vi "Read Msg Input.vi"(11 "Start Msg Input in":refnum<class "Start Msg Input.lvclass">) -> (4 "Teller":refnum<class "Teller.lvclass">)   [LabVIEW 2020, in "jettl.lvlib" / "Start jettl Msg.lvlib" / "Start Msg Input.lvlib" / "Start Msg Input.lvclass"]
doc: "jettl 6.14.1.98\nNathan Davis - Nathan Davis\nCopyright (c) 2026, Nathan Davis\nMIT"
uses:
  Start Msg Input.lvclass
  Teller/Teller.lvclass
  Start Msg Input.lvclass/Start Msg Input.ctl
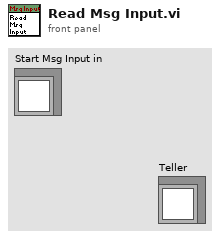
[diagram p1: front panel]
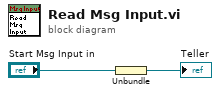
[diagram p0: block diagram]
diagram:
  n1 = Unbundle "Unbundle"("Start Msg Input in") -> (→"Teller":refnum<class "Teller.lvclass">)
